vi "CANFD Set Relay.vi"(10 "RelayState":u8, 11 "DevHandle":i32) -> (3 "function return":i32)   [LabVIEW 2010, in "usb2canfd.lvlib"]
doc: "int WINAPI CANFD_SetRelay(int DevHandle, unsigned char RelayState);"
uses:
  usb2canfd.lvlib
  USB2XXX/trunk/USB2XXX/USB2XXX/vs2019/Release/USB2XXX.dll
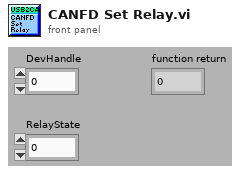
[diagram p1: front panel]
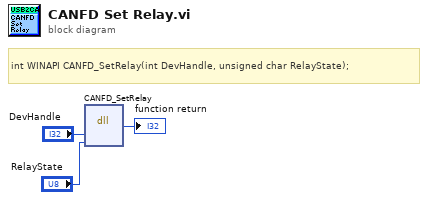
[diagram p0: block diagram]
diagram:
  # "int WINAPI CANFD_SetRelay(int DevHandle, unsigned char RelayState);"
  n1 = dll-call lib="E:/Projects/USB2XXX/trunk/USB2XXX/USB2XXX/vs2019/Release/USB2XXX.*" fn="CANFD_SetRelay"("DevHandle"="DevHandle", "RelayState"="RelayState") -> (→"function return":i32)  [unwired: 5 in, 2 out]
